vi "Demo.vi"() -> ()   [LabVIEW 2022 SP3]
uses:
  Components/ViPER.lvlibp/ViPER.lvclass
panel:
  in  "Config XML":string="<Object>\n<Name>Count</Name>\n<Class>Frequency_Counter_TTi</Class>\n</Object>"
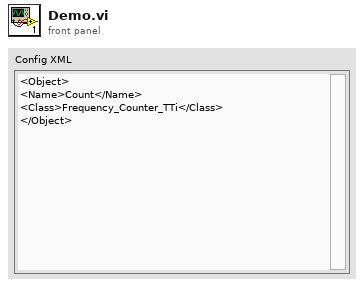
[diagram p1: front panel]
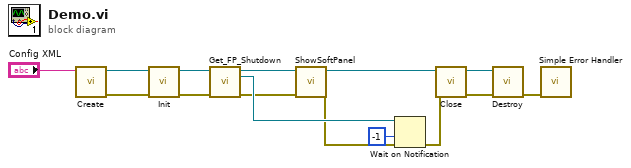
[diagram p0: block diagram]
diagram:
  n1 = call "Create.vi"("Config XML"="Config XML") -> ("error out"=w11:errorcluster, "reference out"=w12:refnum<class "ViPER.lvclass">)  [unwired: 9 in]
  n2 = call-dynamic "Init.vi"("error in (no error)"=w11, "reference in"=w12) -> ("error out"=w9:errorcluster, "reference out"=w10:refnum<class "ViPER.lvclass">)  [unwired: 8 in]
  n3 = call "Get_FP_Shutdown.vi"("ViPER_Base in"=w10, "error in (no error)"=w9) -> ("ViPER_Base out"=w7:refnum<class "ViPER.lvclass">, "SoftFP_Shutdown"=w8:refnum<notifier>, "error out"=w6:errorcluster)  [unwired: 10 in, 1 out]
  n4 = call-dynamic "ShowSoftPanel.vi"("error in (no error)"=w6, "Driver in"=w7) -> ("error out"=w5:errorcluster, "Driver out"=w4:refnum<class "ViPER.lvclass">)  [unwired: 7 in, 1 out]
  n5 = Wait on Notification(notifier=w8, timeout in ms (-1)=-1, error in (no error)=w5) -> (error out=w15:errorcluster)  [unwired: 1 in, 3 out]
  n6 = call-dynamic "Close.vi"("error in (no error)"=w15, "reference in"=w4) -> ("error out"=w3:errorcluster, "reference out"=w1:refnum<class "ViPER.lvclass">)  [unwired: 8 in]
  n7 = call "Destroy.vi"("error in (no error)"=w3, "reference in"=w1) -> ("error out"=w2:errorcluster)  [unwired: 9 in]
  n8 = call <vilib>:"Simple Error Handler.vi"("error in (no error)"=w2) -> ()  [unwired: 4 in, 5 out]
